vi "Bundle.vi"(8 "error in (no error)":errorcluster, 9 "Data Array":refnum<class "Data.lvclass">[](array[class]), 10 "Message Array":refnum<class "Message.lvclass">[](array[class]), 11 "Subscribe Msg in":refnum<class "Subscribe Msg.lvclass">) -> (0 "error out":errorcluster, 3 "Subscribe Msg out":refnum<class "Subscribe Msg.lvclass">)   [LabVIEW 2020, in "Publisher.lvlib" / "Subscribe Msg.lvclass"]
doc: "Populate the Subscribe Msg class."
uses:
  Subscribe Msg.lvclass
  PPL/HDH.Actor Framework.Core.Actor.lvlibp/1abvi3w/vi.lib/ActorFramework/Message/Message.lvclass
  PPL/HDH.Data.Generic.lvlibp/Data.lvclass
  Subscribe Msg.lvclass/Subscribe Msg.ctl
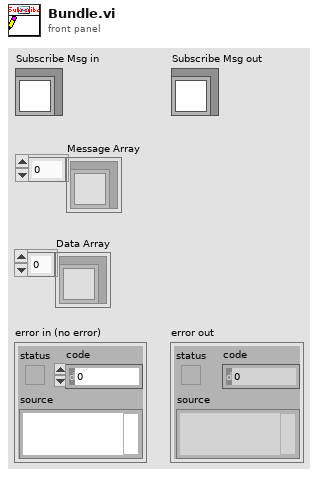
[diagram p1: front panel]
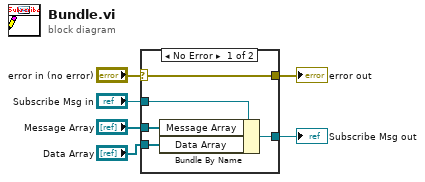
[diagram p0: block diagram]
diagram:
  n1 = case shown="No Error" "error in (no error)" {
    selector: "error in (no error)" -> [w11 w12]
    tunnel: [w11 w12] -> w5
    tunnel: [w9 w13] -> w3
    tunnel: "Subscribe Msg in" -> [w10 w13]
    tunnel: "Message Array" -> [w8 _]
    tunnel: "Data Array" -> [w7 _]
    frame No Error {
      n2 = Bundle By Name(cluster=w10, "Message Array"=w8, "Data Array"=w7) -> (w9:refnum<class "Subscribe Msg.lvclass">)
    }
    frame Error {
    }
  }
  "error out" <- w5
  "Subscribe Msg out" <- w3
